vi "Create Workbook.vi"(7 "Worksheet Format (XLSX)":T1, 10 "Sheetname (Sheet1)":string="Sheet1", 11 "File Name":path=path "C:/PhaeronGit/LVNPOI/Scratch/test.xls") -> (0 "error out":errorcluster, 2 "Sheet Reference":refnum<k24>, 3 "IWorkbook Reference":refnum<k24>)   [LabVIEW 2014]
uses:
  C:/Users/LENOVO/Desktop/CodeSpace GUI/LVExcel/Resources/NPOI.dll
  Resources/NPOI.dll
  Typedefs/Worksheet Format.ctl
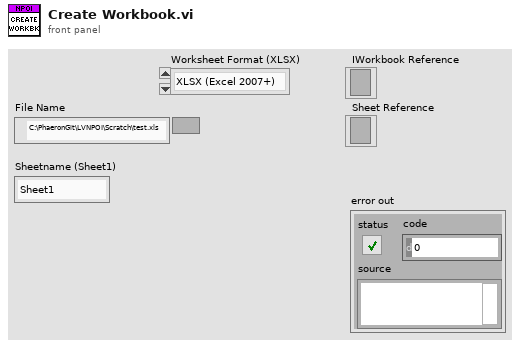
[diagram p1: front panel]
types:
  T1 = typedef "Worksheet Format.ctl" = enum16{"XLSX (Excel 2007+)", "XLS (Excel Legacy)"}
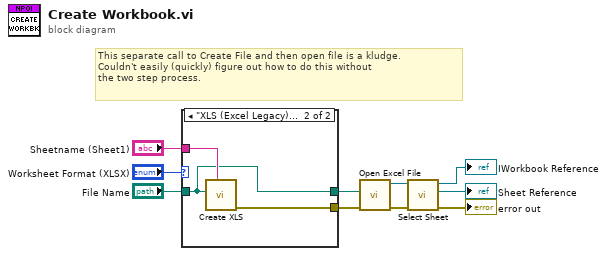
[diagram p0: block diagram]
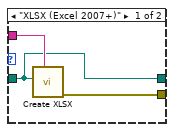
[diagram p2: hidden frame]
diagram:
  # "This separate call to Create File and then open file is a kludge.\nCouldn't easily (quickly) figure out how to do this without\nthe two step process."
  n1 = case shown="\"XLS (Excel Legacy)\"" "Worksheet Format (XLSX)" {
    tunnel: "File Name" -> [w11 w14]
    tunnel: "Sheetname (Sheet1)" -> [w13 w16]
    tunnel: [w12 w15] -> w7
    tunnel: [w11 w14] -> w6
    frame "XLSX (Excel 2007+)" {
      n2 = call "Create XLSX.vi"("sheetname"=w13, "File Name"=w11) -> ("error out"=w12:errorcluster)  [unwired: 9 in]
    }
    frame "XLS (Excel Legacy)" {
      n3 = call "Create XLS.vi"("sheetname"=w16, "File Name"=w14) -> ("error out"=w15:errorcluster)  [unwired: 9 in]
    }
  }
  n4 = call "Open Excel File.vi"("error in (no error)"=w7, "File Name"=w6) -> ("error out"=w5:errorcluster, "IWorkbook Reference Out"=w4:refnum<k24>)  [unwired: 8 in]
  n5 = call "Select Sheet.vi"("error in (no error)"=w5, "IWorkbook Reference"=w4) -> ("error out"=→"error out":errorcluster, "Sheet Reference"=→"Sheet Reference":refnum<k24>, "IWorkbook Reference"=→"IWorkbook Reference":refnum<k24>)  [unwired: 7 in]
